vi "Signal setting generator.vi"(6 "rate":dbl, 7 "Vx_Max":dbl, 8 "N_y":i32, 9 "N_x":i32, 10 "Ratio":dbl, 11 "Vy_Max":dbl) -> (3 "Waveform out":T1)   [LabVIEW 2013]
doc: "输出整合后的<b>标准采样模式簇<\\b>"
panel:
  # "IN"
  # "OUT"
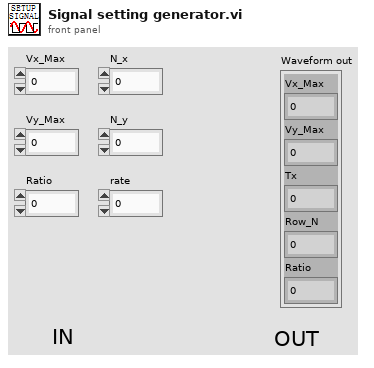
[diagram p1: front panel]
types:
  T1 = cluster{"Vx_Max":dbl, "Vy_Max":dbl, "Tx":dbl, "Row_N":i32, "Ratio":dbl}
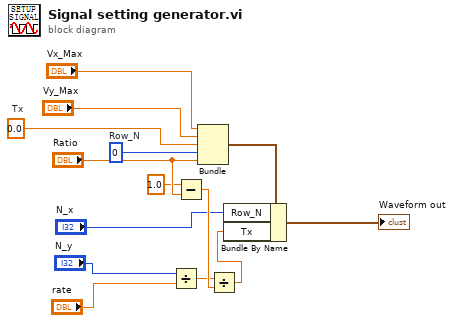
[diagram p0: block diagram]
diagram:
  w2 = 0.0  # Tx
  w8 = 0  # Row_N
  n1 = Divide(x="N_y", y="rate") -> (x/y=w10:dbl)
  n2 = Subtract(x=1.0, y="Ratio") -> (x-y=w13:dbl)
  n3 = Bundle("Vx_Max"="Vx_Max", "Vy_Max"="Vy_Max", "Tx"=w2, "Row_N"=w8, "Ratio"="Ratio") -> (w9:T1)  [unwired: 1 in]
  n4 = Divide(x=w10, y=w13) -> (x/y=w14:dbl)
  n5 = Bundle By Name(cluster=w9, "Row_N"="N_x", "Tx"=w14) -> (→"Waveform out":T1)
